vi "2DSketch.vi"(8 "Setup":T2={"Scaling (pixels/mm)"=1.0, "Tool Diameter (inch)"=0.25, "Origin location"={"x (mm)"=10, "y (mm)"=300}, "Wood dim"={"width (inch)"=10.0, "height (inch)"=300.0}}, 11 "cmd amd State":cluster{"Command":string, "End State":dbl[]}[](array[cluster])) -> (1 "Bounds":T1 {"Z Max" format="%#.1f"; "Z Min" format="%#.1f"; "Y Max" format="%#.1f"; "Y Min" format="%#.1f"; "X Max" format="%#.1f"; "X Min" format="%#.1f"}, 3 "Cut":picture)   [LabVIEW 2023]
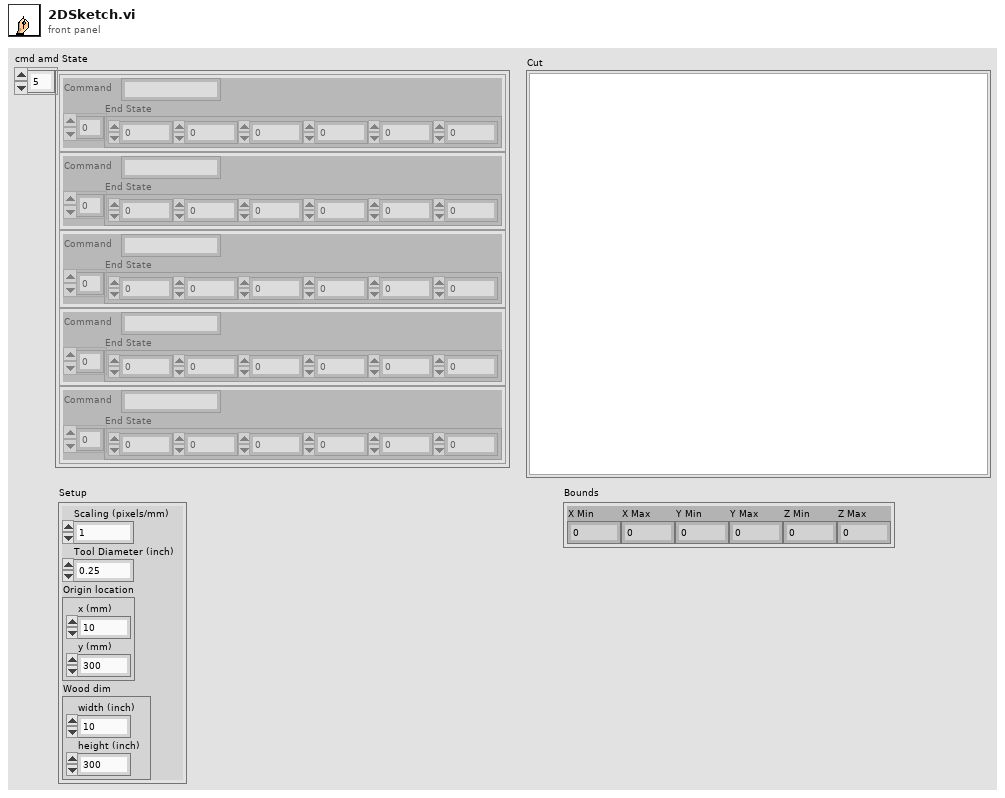
[diagram p1: front panel]
types:
  T1 = cluster{"X Min":dbl, "X Max":dbl, "Y Min":dbl, "Y Max":dbl, "Z Min":dbl, "Z Max":dbl}
  T2 = cluster{"Scaling (pixels/mm)":dbl, "Tool Diameter (inch)":dbl, "Origin location":cluster{"x (mm)":i16, "y (mm)":i16}, "Wood dim":cluster{"width (inch)":dbl, "height (inch)":dbl}}
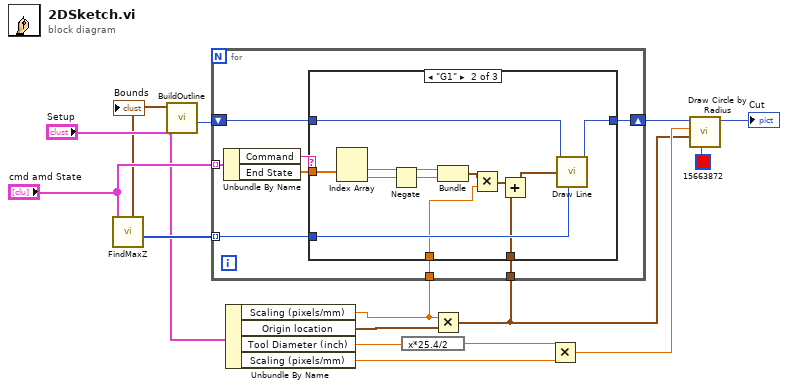
[diagram p0: block diagram]
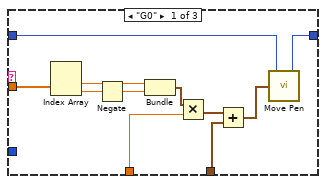
[diagram p2: hidden frame]
diagram:
  n1 = call "FindMaxZ.vi"("cmd amd State"="cmd amd State") -> ("Z Colors"=w11:u32[], "Cutting Bounds"=w1:T1)  [unwired: 7 in, 2 out]
  "Bounds" <- w1
  n2 = call "BuildOutline.vi"("Setup"="Setup", "Bounds"=w1) -> ("new picture"=w2:picture)  [unwired: 8 in, 1 out]
  n3 = Unbundle By Name("Setup") -> ("Scaling (pixels/mm)"=w5:dbl, "Origin location"=w4:cluster{"x (mm)":i16, "y (mm)":i16}, "Tool Diameter (inch)"=w10:dbl, "Scaling (pixels/mm)"=w9:dbl)
  n4 = expression code="x*25.4/2"(w10) -> (w8:dbl)
  n5 = Multiply(x=w5, y=w4) -> (x*y=w6:cluster{"x (mm)":dbl, "y (mm)":dbl})
  n6 = for {
    shift-right: [w22] -> w15
    shift-left: w2 -> [w23]
    tunnel: "cmd amd State" -> [w21] mode=indexing
    tunnel: w6 -> [w18]
    tunnel: w11 -> [w17] mode=indexing
    tunnel: w5 -> [w16]
    n7 = Unbundle By Name(w21) -> ("Command"=w20:string, "End State"=w19:dbl[])
    n8 = case shown="\"G1\"" w20 {
      tunnel: w23 -> [w34 w46 w47]
      tunnel: [w33 w45 w47] -> w22
      tunnel: w19 -> [w30 w42 _]
      tunnel: w18 -> [w29 w35 _]
      tunnel: w17 -> [_ w39 _]
      tunnel: w16 -> [w26 w36 _]
      frame "G0" {
        n9 = Index Array(array=w30) -> (element #1=w32:dbl, element #2=w31:dbl)  [unwired: 2 in]
        n10 = Negate(x=w31) -> (-x=w27:dbl)
        n11 = Bundle(w32, w27) -> (w25:cluster{dbl, dbl})  [unwired: 1 in]
        n12 = Multiply(x=w25, y=w26) -> (x*y=w24:cluster{dbl, dbl})
        n13 = Add(x=w24, y=w29) -> (x+y=w28:cluster{dbl, dbl})
        n14 = call <vilib>:"Move Pen.vi"("new position"=w28, "picture"=w34) -> ("new picture"=w33:picture)  [unwired: 3 in]
      }
      frame "G1" {
        n15 = Index Array(array=w42) -> (element #1=w44:dbl, element #2=w43:dbl)  [unwired: 2 in]
        n16 = Negate(x=w43) -> (-x=w40:dbl)
        n17 = Bundle(w44, w40) -> (w38:cluster{dbl, dbl})  [unwired: 1 in]
        n18 = Multiply(x=w38, y=w36) -> (x*y=w37:cluster{dbl, dbl})
        n19 = Add(x=w37, y=w35) -> (x+y=w41:cluster{dbl, dbl})
        n20 = call <vilib>:"Draw Line.vi"("picture"=w46, "end point"=w41, "color(black)"=w39) -> ("new picture"=w45:picture)  [unwired: 6 in]
      }
      frame Default {
      }
    }
  }
  n21 = Multiply(x=w8, y=w9) -> (x*y=w7:dbl)
  n22 = call <vilib>:"Draw Circle by Radius.vi"("color(black)"=u32 15663872, "pixel center"=w6, "radius"=w7, "picture"=w15) -> ("new picture"=→"Cut":picture)  [unwired: 7 in]
